vi "generate filepath.vi"(1 "Filename":string, 2 "Subfolder(no outside slashes)":string, 3 "Prepend date folder?":bool, 4 "Scan base":path=path "T:/Physics/Minot Group/Lee/SPCM/SPCM Setup/stringtest/scan") -> (0 "path":path)   [LabVIEW 2013]
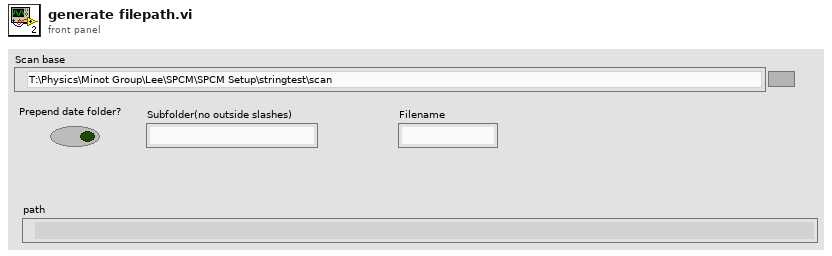
[diagram p1: front panel]
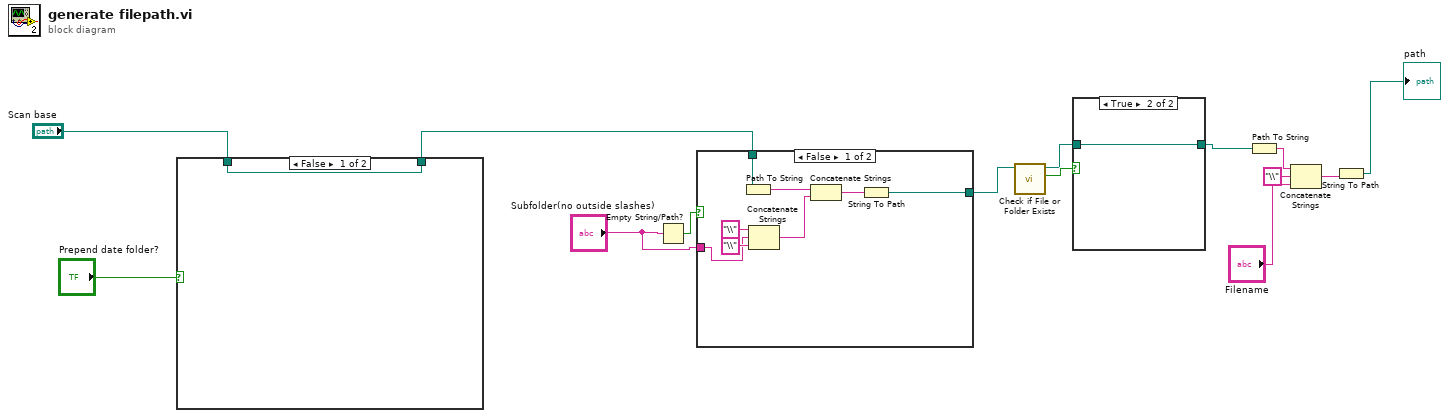
[diagram p0: block diagram]
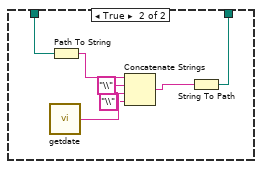
[diagram p2: hidden frame]
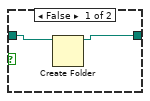
[diagram p4: hidden frame]
diagram:
  n1 = case shown="False" "Prepend date folder?" {
    tunnel: "Scan base" -> [w15 w22]
    tunnel: [w15 w16] -> w1
    frame False {
    }
    frame True {
      n2 = call "getdate.vi"() -> ("date/time string"=w19:string)  [unwired: 1 in]
      n3 = Path To String(path=w22) -> (string=w21:string)
      n4 = Concatenate Strings(w21, "\\" ("string"), w19, "\\" ("string")) -> (w17:string)
      n5 = String To Path(string=w17) -> (path=w16:path)
    }
  }
  n6 = Empty String/Path?(string/path="Subfolder(no outside slashes)") -> (empty?=w5:bool)
  n7 = case shown="False" w5 {
    tunnel: w1 -> [w30 w31]
    tunnel: [w24 w31] -> w14
    tunnel: "Subfolder(no outside slashes)" -> [w23 _]
    frame False {
      n8 = Path To String(path=w30) -> (string=w29:string)
      n9 = Concatenate Strings("\\" ("string"), w23, "\\" ("string")) -> (w26:string)
      n10 = Concatenate Strings(w29, w26) -> (w25:string)
      n11 = String To Path(string=w25) -> (path=w24:path)
    }
    frame True {
    }
  }
  n12 = call <vilib>:"Check if File or Folder Exists.vi"("path"=w14) -> ("file or folder exists?"=w13:bool, "dup path"=w12:path)  [unwired: 8 in, 1 out]
  n13 = case shown="True" w13 {
    tunnel: w12 -> [w33 w34]
    tunnel: [w32 w34] -> w11
    frame False {
      n14 = Create Folder(path (use dialog)=w33) -> (created path=w32:path)  [unwired: 2 in, 2 out]
    }
    frame True {
    }
  }
  n15 = Path To String(path=w11) -> (string=w10:string)
  n16 = Concatenate Strings(w10, "\\" ("string"), "Filename") -> (w8:string)
  n17 = String To Path(string=w8) -> (path=→"path":path)
